vi "SonarGetRange.vi"() -> (3 "Distance":dbl)   [LabVIEW 2015]
uses:
  <vilib>/Rock Robotics/WPI/Ultrasonic/WPI_SonarMB1010AnalogRefNum Registry Get.vi
  <vilib>/Rock Robotics/WPI/Ultrasonic/WPI_SonarMB1010AnalogGetRange.vi
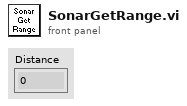
[diagram p1: front panel]
types:
  T1 = typedef "WPI_SonarMB1010AnalogDeviceRef.ctl" = cluster{"AIDeviceRef":T2, "Scaling factor (V/in)":dbl, "Average Bits":u8}
  T2 = typedef "WPI_AnalogChannelDevRef.ctl" = cluster{"DevStatus":errorcluster, "Analog Channel":T3}
  T3 = typedef "FPGA_AIChannel.ctl" = enum8{"AI 0", "AI 1", "AI 2", "AI 3", "AI MXP 0", "AI MXP 1", "AI MXP 2", "AI MXP 3", "Invalid"}
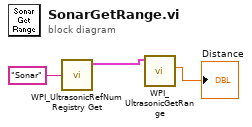
[diagram p0: block diagram]
diagram:
  n1 = call-poly <vilib>:"WPI_UltrasonicRefNum Registry Get.vi"("refnum name"="Sonar") -> ("SonarMB1010AnalogDevRef"=w2:T1)  [unwired: 9 in, 1 out]
  n2 = call-poly <vilib>:"WPI_UltrasonicGetRange.vi"("SonarMB1010AnalogDevRef"=w2) -> ("Distance"=→"Distance":dbl)  [unwired: 8 in, 2 out]
